vi "Set Editor Position.vi"(7 "IE VI Ref":refnum<vi>, 8 "error in":errorcluster, 9 "Use Size":bool, 10 "Bounds Vaid":bool, 11 "Window Bounds":T1) -> (0 "error out":errorcluster)   [LabVIEW 2020, in "lv_icon.lvlib"]
doc: "Reads the position from the LabVIEW INI file and sets the position of the editor. If the INI token is missing or formatted incorrectly, the editor will be centered on the caller's monitor."
uses:
  vi.lib/LabVIEW Icon API/lv_icon/lv_icon.lvlib
  <vilib>/Utility/miscctls.llb/LVRectTypeDef.ctl
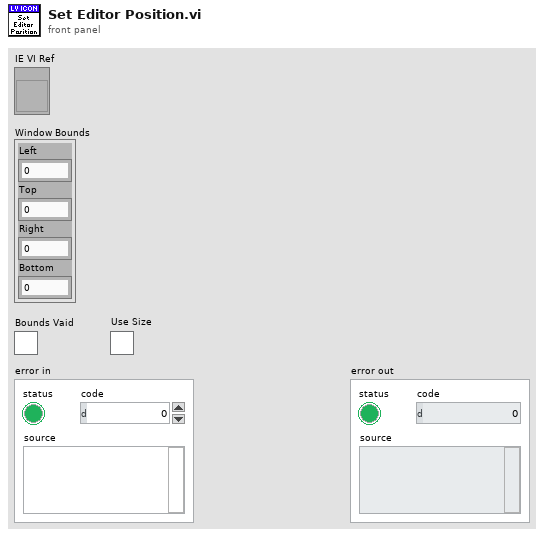
[diagram p1: front panel]
types:
  T1 = typedef "LVRectTypeDef.ctl" = cluster{"Left":i16, "Top":i16, "Right":i16, "Bottom":i16}
  T2 = typedef "LVAllMonitorsDisplayTypeDef.ctl" = cluster{"Bounds":cluster{"Left":i16, "Top":i16, "Right":i16, "Bottom":i16}, "Depth":i16}[]
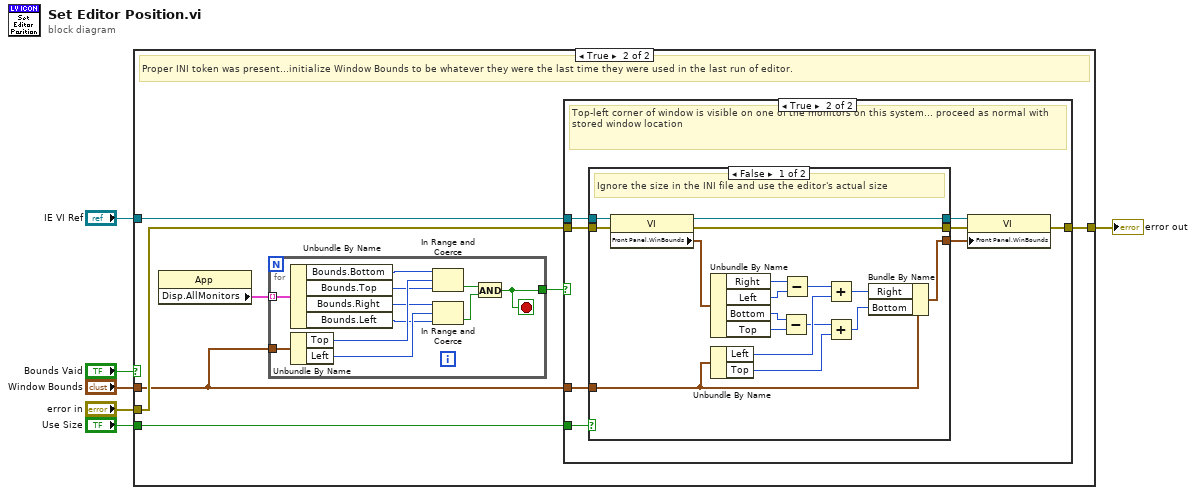
[diagram p0: block diagram]
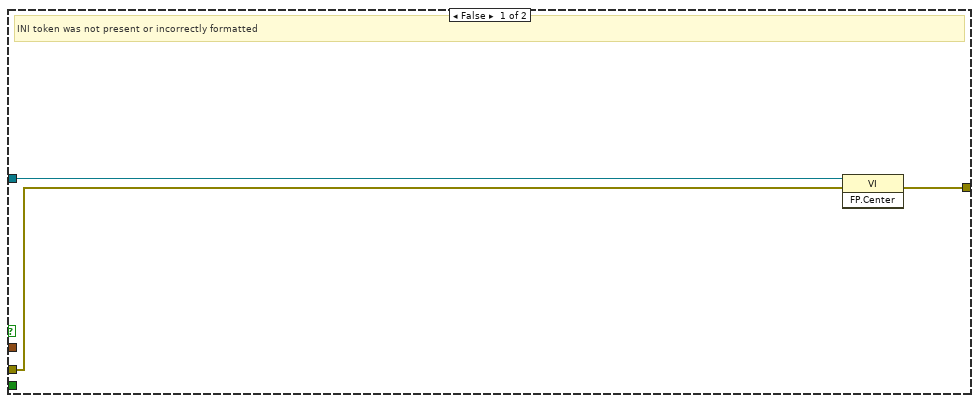
[diagram p2: hidden frame]
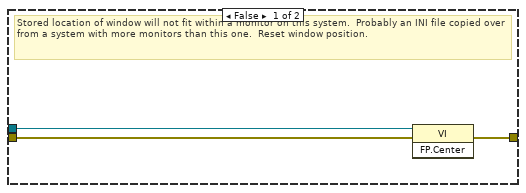
[diagram p3: hidden frame]
diagram:
  n1 = case shown="True" "Bounds Vaid" {
    tunnel: "Use Size" -> [_ w10]
    tunnel: "IE VI Ref" -> [w7 w11]
    tunnel: [w9 w16] -> w6
    tunnel: "error in" -> [w8 w15]
    tunnel: "Window Bounds" -> [_ w12]
    frame False {
      # "INI token was not present or incorrectly formatted"
      n2 = invoke class="VI" method="FP.Center"(reference=w7, error in=w8) -> (error out=w9:errorcluster)  [unwired: 1 in, 2 out]
    }
    frame True {
      # "Proper INI token was present...initialize Window Bounds to be whatever they were the last time they were used in the last run of editor."
      n3 = property class="App"() -> ("Disp.AllMonitors"=w14:T2)  [unwired: 2 in, 2 out]
      n4 = for {
        tunnel: w14 -> [w56] mode=indexing
        tunnel: [w49] -> w13
        tunnel: w12 -> [w48]
        stop <- w49 stop-if-true
        n5 = Unbundle By Name(w56) -> ("Bounds.Bottom"=w52:i16, "Bounds.Top"=w53:i16, "Bounds.Right"=w55:i16, "Bounds.Left"=w54:i16)
        n6 = Unbundle By Name(w48) -> ("Top"=w57:i16, "Left"=w58:i16)
        n7 = In Range and Coerce(upper limit=w52, x=w57, lower limit=w53) -> (In Range?=w51:bool)  [unwired: 1 out]
        n8 = In Range and Coerce(upper limit=w55, x=w58, lower limit=w54) -> (In Range?=w50:bool)  [unwired: 1 out]
        n9 = And(x=w51, y=w50) -> (x .and. y?=w49:bool)
      }
      n10 = case shown="True" w13 {
        tunnel: w12 -> [_ w22]
        tunnel: w11 -> [w17 w24]
        tunnel: w15 -> [w19 w26]
        tunnel: [w18 w27] -> w16
        tunnel: w10 -> [_ w21]
        frame False {
          # "Stored location of window will not fit within a monitor on this system.  Probably an INI file copied over from a system with more monitors than this one.  Reset window position."
          n11 = invoke class="VI" method="FP.Center"(reference=w17, error in=w19) -> (error out=w18:errorcluster)  [unwired: 1 in, 2 out]
        }
        frame True {
          # "Top-left corner of window is visible on one of the monitors on this system... proceed as normal with stored window location"
          n12 = case shown="False" w21 {
            tunnel: w24 -> [w42 w46]
            tunnel: w26 -> [w44 w47]
            tunnel: [w36 w46] -> w23
            tunnel: [w43 w47] -> w25
            tunnel: w22 -> [w31 w45]
            tunnel: [w28 w45] -> w20
            frame False {
              # "Ignore the size in the INI file and use the editor's actual size"
              n13 = property class="VI"(reference=w42, error in=w44) -> (reference out=w36:refnum<vi>, error out=w43:errorcluster, "Front Panel.WinBounds"=w41:T1)
              n14 = Unbundle By Name(w41) -> ("Right"=w40:i16, "Left"=w39:i16, "Bottom"=w38:i16, "Top"=w37:i16)
              n15 = Unbundle By Name(w31) -> ("Left"=w34:i16, "Top"=w32:i16)
              n16 = Subtract(x=w38, y=w37) -> (x-y=w33:i16)
              n17 = Subtract(x=w40, y=w39) -> (x-y=w35:i16)
              n18 = Add(x=w35, y=w34) -> (x+y=w30:i16)
              n19 = Add(x=w33, y=w32) -> (x+y=w29:i16)
              n20 = Bundle By Name(cluster=w31, "Right"=w30, "Bottom"=w29) -> (w28:T1)
            }
            frame True {
              # "Token set to use the position size"
            }
          }
          n21 = property class="VI"(reference=w23, error in=w25, "Front Panel.WinBounds"=w20) -> (error out=w27:errorcluster)  [unwired: 1 out]
        }
      }
    }
  }
  "error out" <- w6
